vi "VI_SetChList.vi"(8 "error in (no error)":errorcluster, 10 "Channel List":cluster{"ID":string, "Name":string}[](array[cluster]), 11 "ChList_Ref In":refnum<vi>) -> (0 "error out":errorcluster, 3 "ChList_Ref Out":refnum<vi>)   [LabVIEW 2018]
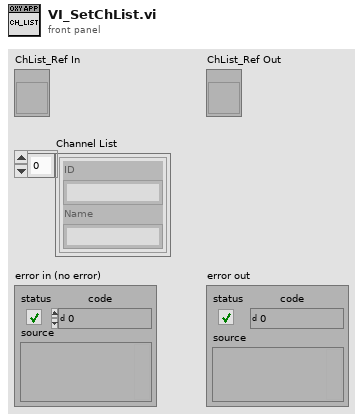
[diagram p1: front panel]
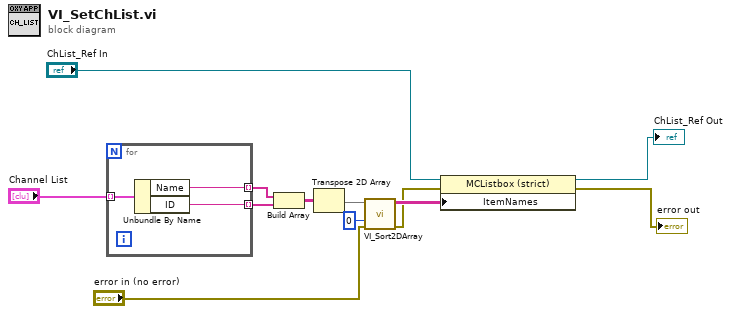
[diagram p0: block diagram]
diagram:
  n1 = for {
    tunnel: "Channel List" -> [w15] mode=indexing
    tunnel: [w14] -> w8 mode=indexing
    tunnel: [w13] -> w7 mode=indexing
    n2 = Unbundle By Name(w15) -> ("Name"=w14:string, "ID"=w13:string)
  }
  n3 = Build Array(w8, w7) -> (w6:string[][])
  n4 = Transpose 2D Array(2D array=w6) -> (transposed array=w5:string[][])
  n5 = call "VI_Sort2DArray.vi"("error in (no error)"="error in (no error)", "Collumn to sort by"=i16 0, "Array In"=w5) -> ("error out"=w2:errorcluster, "Array Out"=w3:string[][])  [unwired: 7 in]
  n6 = property class="MCListbox (strict)"(reference="ChList_Ref In", error in=w2, "ItemNames"=w3) -> (reference out=→"ChList_Ref Out":refnum<vi>, error out=→"error out":errorcluster)
